vi "MW_Set Power(dBm).vi"(8 "错误输入（无错误）":errorcluster, 10 "Power (dBm)":dbl, 11 "VISA引用句柄输入":refnum<visa-resource-name>) -> (0 "错误输出":errorcluster, 2 "Command":string, 3 "VISA引用句柄输出":refnum<visa-resource-name>)   [LabVIEW 2016, in "Microwave Source.lvlib"]
doc: "设置微波源输出功率。"
uses:
  Microwave Source.lvlib
panel:
  out "read buffer":string
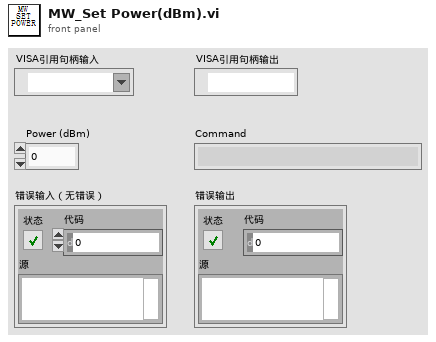
[diagram p1: front panel]
types:
  T1 = typedef "Microwave Source.lvlib/MW_ctl_DeviceType.ctl" = enum16{"R&S", "Other"}
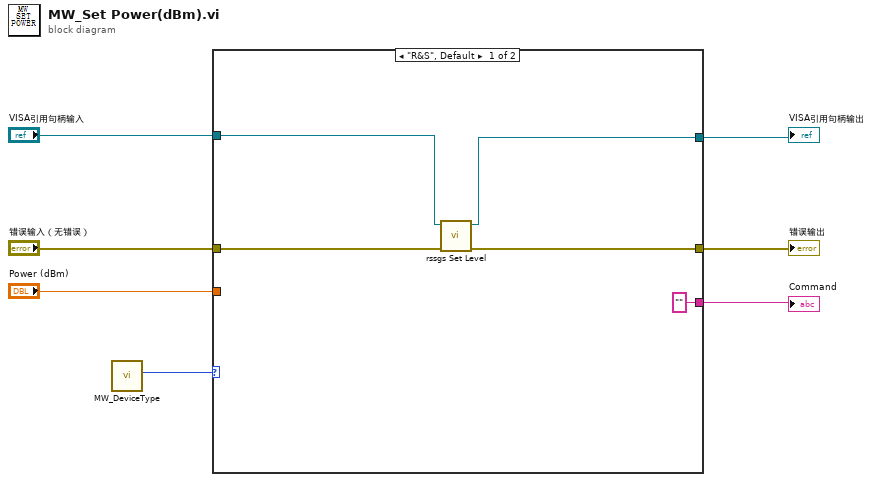
[diagram p0: block diagram]
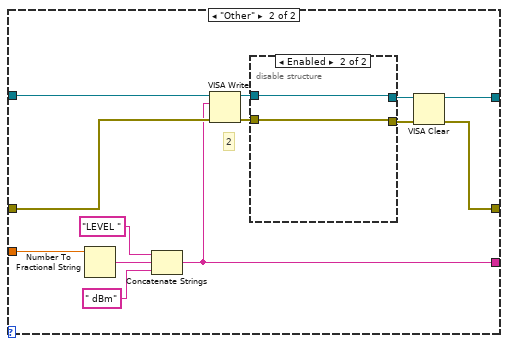
[diagram p2: hidden frame]
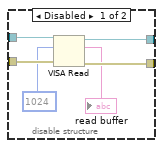
[diagram p3: hidden frame]
diagram:
  n1 = call "MW_DeviceType.vi"() -> ("DeviceType"=w1:T1)  [unwired: 11 in]
  n2 = case shown="\"R&S\", Default" w1 {
    tunnel: "错误输入（无错误）" -> [w10 w25]
    tunnel: "VISA引用句柄输入" -> [w12 w24]
    tunnel: ["" w23] -> w5
    tunnel: "Power (dBm)" -> [_ w19]
    tunnel: [w9 w14] -> w3
    tunnel: [w11 w13] -> w2
    frame "R&S", Default {
      n3 = call <instrlib>:"rssgs Set Level.vi"("error in (no error)"=w10, "VISA resource name"=w12) -> ("error out"=w9:errorcluster, "VISA resource name out"=w11:refnum<visa-resource-name>)  [unwired: 8 in]
    }
    frame "Other" {
      # "2"
      n4 = Number To Fractional String(number=w19) -> (F-format string=w20:string)  [unwired: 3 in]
      n5 = Concatenate Strings("LEVEL ", w20, " dBm") -> (w23:string)
      n6 = VISA Write(VISA resource name=w24, write buffer=w23, error in (no error)=w25) -> (VISA resource name out=w17:refnum<visa-resource-name>, error out=w18:errorcluster)  [unwired: 1 out]
      n7 = disable-structure shown="Enabled" {
        disable-tunnel: w18 -> [w31 w32]
        disable-tunnel: w17 -> [w30 w33]
        disable-tunnel: [w28 w32] -> w16
        disable-tunnel: [w27 w33] -> w15
        frame Disabled {
          n8 = VISA Read(VISA resource name=w30, byte count=u32 1024, error in (no error)=w31) -> (VISA resource name out=w27:refnum<visa-resource-name>, read buffer=→"read buffer":string, error out=w28:errorcluster)  [unwired: 1 out]
        }
        frame Enabled {
        }
      }
      n9 = VISA Clear(VISA resource name=w15, error in (no error)=w16) -> (VISA resource name out=w13:refnum<visa-resource-name>, error out=w14:errorcluster)
    }
  }
  "VISA引用句柄输出" <- w2
  "错误输出" <- w3
  "Command" <- w5
